vi "滤波模块.vi"(7 "首次调用":bool, 9 "通量in":dbl[](array[numeric])) -> (1 "滤波开":bool, 3 "通量out":dbl[](array[numeric]))   [LabVIEW 2020]
uses:
  <vilib>/Analysis/3filter.llb/Savitzky-Golay Filter (DBL).vi
  <vilib>/Analysis/3filter.llb/FIR Filter (DBL).vi
  <vilib>/Analysis/NI_AALBase.lvlib
panel:
  in  "滤波数组":dbl[][](array[numeric])
  in  "上一点":dbl[](array[numeric])
  in  "滤波显示选择":u16(ring) caption="滤波显示选择：" items=["电流1", "电流2"]
  in  "滤波方法选择":T1(tab) caption="滤波方法选择："
  in  "滤波系数(0-0.99):":dbl=0.5 min=0.0 max=0.99 step=0.01 format="%#.2f"
  in  "左秩:":i32
  in  "side points":i32=24 caption="单侧数据点数:"
  in  "polynomial":i32=3 caption="多项式阶数:"
  in  "滤波系数：":dbl=0.1
  in  "滤波点数：":i32=10
  in  "开关":bool caption="滤波开关："
  in  "通量名称":string[](array[string])
  out "滤波效果图":dbl[][](graph) caption="滤波效果图："
  # "0相位滤波"
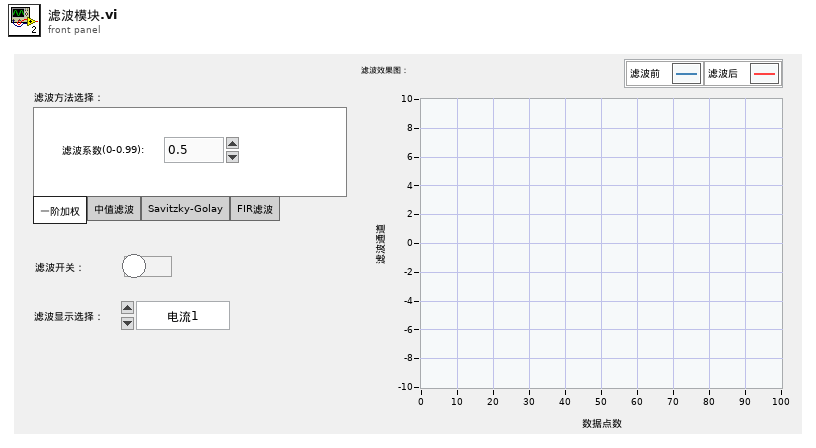
[diagram p1: front panel]
types:
  T1 = enum32{"一阶加权", "中值滤波", "Savitzky-Golay", "FIR滤波"}
  T2 = enum8{"Enabled", "Disabled", "Disabled and Grayed Out"}
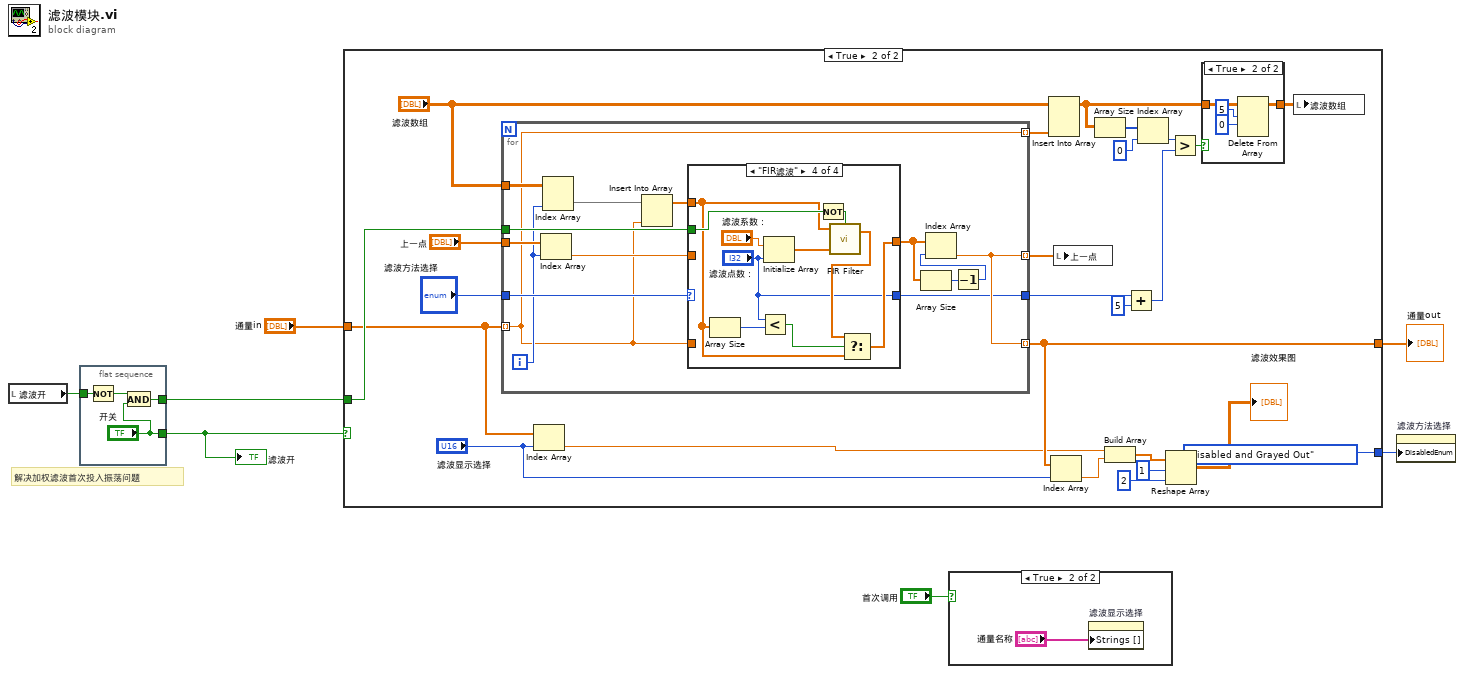
[diagram p0: block diagram]
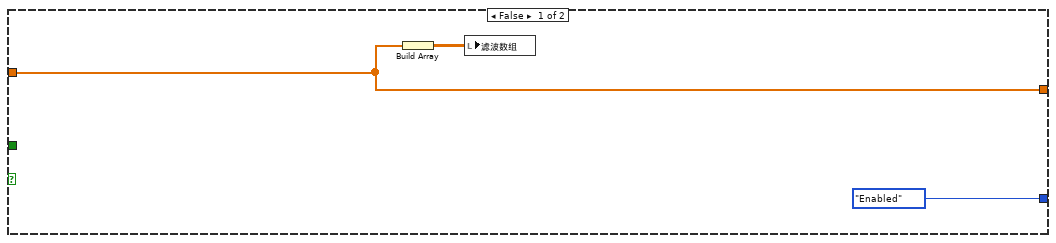
[diagram p2: hidden frame]
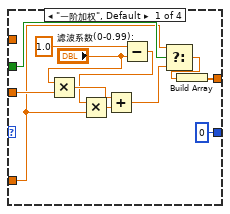
[diagram p4: hidden frame]
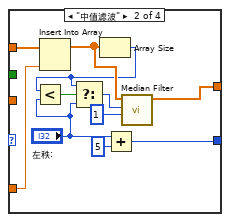
[diagram p5: hidden frame]
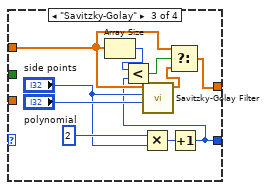
[diagram p6: hidden frame]
diagram:
  # "解决加权滤波首次投入振荡问题"
  n1 = local read "滤波开"() -> (w5:bool)
  n2 = flat-sequence {
    tunnel: ["开关"] -> w7
    tunnel: [w9] -> w6
    tunnel: w5 -> [w8]
    frame #0 {
      n3 = Not(x=w8) -> (.not. x?=w11:bool)
      n4 = And(x=w11, y="开关") -> (x .and. y?=w9:bool)
    }
  }
  n5 = case shown="True" w7 {
    tunnel: "通量in" -> [w12 w37]
    tunnel: [w12 w36] -> w2
    tunnel: w6 -> [_ w38]
    tunnel: [T2."Enabled" ("禁用") T2."Disabled and Grayed Out" ("禁用")] -> w4
    frame False {
      n6 = Build Array(w12) -> (w13:dbl[][])
      n7 = local write "滤波数组"(w13) -> ()
    }
    frame True {
      n8 = for {
        tunnel: "滤波方法选择" -> [w58]
        tunnel: w38 -> [w57]
        tunnel: w37 -> [w49] mode=indexing
        tunnel: [w54] -> w36 mode=indexing
        tunnel: [w54] -> w26 mode=indexing
        tunnel: "上一点" -> [w56]
        tunnel: [w49] -> w25 mode=indexing
        tunnel: "滤波数组" -> [w53]
        tunnel: [w50] -> w23
        i -> [w52]
        n9 = Index Array(array=w56, index=w52) -> (element=w55:dbl)
        n10 = Index Array(array=w53, index (col)=w52) -> (element=w51:dbl[])  [unwired: 1 in]
        n11 = Insert Into Array(array=w51, new element=w49) -> (w45:dbl[])  [unwired: 1 in]
        n12 = case shown="\"FIR滤波\"" w58 {
          tunnel: w49 -> [w59 w80 _ _]
          tunnel: w57 -> [w62 _ _ w99]
          tunnel: w55 -> [w65 _ _ _]
          tunnel: w45 -> [_ w81 w86 w96]
          tunnel: [w64 w74 w88 w97] -> w46
          tunnel: [0 w72 w82 "滤波点数："] -> w50
          frame "一阶加权", Default {
            n13 = Multiply(x="滤波系数(0-0.99):", y=w65) -> (x*y=w68:dbl)
            n14 = Subtract(x=1.0 ("新点权重%"), y="滤波系数(0-0.99):") -> (x-y=w66:dbl)
            n15 = Multiply(x=w66, y=w59) -> (x*y=w69:dbl)
            n16 = Add(x=w68, y=w69) -> (x+y=w60:dbl)
            n17 = Select(t=w59, s=w62, f=w60) -> (s? t:f=w61:dbl)
            n18 = Build Array(w61) -> (w64:dbl[])
          }
          frame "中值滤波" {
            n19 = Insert Into Array(array=w81, new element=w80) -> (w79:dbl[])  [unwired: 1 in]
            n20 = Array Size(array=w79) -> (size(s)=w75:i32)
            n21 = Less?(x=w75, y="左秩:") -> (x < y?=w78:bool)
            n22 = Select(t=w75, s=w78, f="左秩:") -> (s? t:f=w76:i32)
            n23 = Add(x="左秩:", y=5) -> (x+y=w72:i32)
            n24 = call <vilib>:"Median Filter.vi"("right rank"=1, "left rank"=w76, "X"=w79) -> ("Filtered X"=w74:dbl[])  [unwired: 7 in, 1 out]
          }
          frame "Savitzky-Golay" {
            n25 = Array Size(array=w86) -> (size(s)=w85:i32)
            n26 = Multiply(x=2, y="side points") -> (x*y=w89:i32)
            n27 = call-poly <vilib>:"Savitzky-Golay Filter.vi"("polynomial order"="polynomial", "side points"="side points", "X"=w86) -> ("Filtered X"=w87:dbl[])  [unwired: 7 in, 1 out]
            n28 = Increment(x=w89) -> (x+1=w82:i32)
            n29 = Less?(x=w85, y=w82) -> (x < y?=w83:bool)
            n30 = Select(t=w86, s=w83, f=w87) -> (s? t:f=w88:dbl[])
          }
          frame "FIR滤波" {
            n31 = Array Size(array=w96) -> (size(s)=w93:i32)
            n32 = Less?(x="滤波点数：", y=w93) -> (x < y?=w95:bool)
            n33 = Initialize Array("滤波系数：", "滤波点数：") -> (w100:dbl[])
            n34 = Not(x=w99) -> (.not. x?=w92:bool)
            n35 = call-poly <vilib>:"FIR Filter.vi"("init/cont (init:F)"=w92, "FIR Coefficients"=w100, "X"=w96) -> ("Filtered X"=w98:dbl[])  [unwired: 1 in, 1 out]
            n36 = Select(t=w98, s=w95, f=w96) -> (s? t:f=w97:dbl[])
          }
        }
        n37 = Array Size(array=w46) -> (size(s)=w48:i32)
        n38 = Decrement(x=w48) -> (x-1=w47:i32)
        n39 = Index Array(array=w46, index=w47) -> (element=w54:dbl)
      }
      n40 = Index Array(array=w37, index="滤波显示选择") -> (element=w34:dbl)
      n41 = Insert Into Array(array="滤波数组", new element=w25) -> (w30:dbl[][])  [unwired: 2 in]
      n42 = Index Array(array=w36, index="滤波显示选择") -> (element=w19:dbl)
      n43 = local write "上一点"(w26) -> ()
      n44 = Array Size(array=w30) -> (size(s)=w33:i32[])
      n45 = Build Array(w34, w19) -> (w18:dbl[])
      n46 = Add(x=w23, y=5) -> (x+y=w21:i32)
      n47 = Index Array(array=w33, index=0 ("索引")) -> (element=w31:i32)
      n48 = Reshape Array(w18, 1 ("dimension size"), 2 ("dimension size")) -> (→"滤波效果图":dbl[][])
      n49 = Greater?(x=w31, y=w21) -> (0:w29:bool)
      n50 = case shown="True" w29 {
        tunnel: w30 -> [w40 w44]
        tunnel: [w40 w41] -> w28
        frame False {
        }
        frame True {
          n51 = Delete From Array(array=w44, length=5 ("长度"), index (row)=0 ("索引 (行)")) -> (array with subset deleted=w41:dbl[][])  [unwired: 1 in, 1 out]
        }
      }
      n52 = local write "滤波数组"(w28) -> ()
    }
  }
  "通量out" <- w2
  n53 = case shown="True" "首次调用" {
    frame False {
    }
    frame True {
      n54 = property on="滤波显示选择" class="Ring (strict)"("Strings []"="通量名称") -> ()  [unwired: 2 in, 2 out]
    }
  }
  n55 = property on="滤波方法选择" class="TabCtl (strict)"("DisabledEnum"=w4) -> ()  [unwired: 2 in, 2 out]
  "滤波开" <- w7
